vi "SetParam.vi"(8 "error in (no error)":errorcluster caption="entrée d'erreur (pas d'erreur)", 10 "KNNImputer":T1={"missing_values"="nan", "n_neighbors"=5, "weights"="uniform", "metric"="nan_euclidean", "copy"=TRUE, "add_indicator"=FALSE}, 11 "KNNImputer.lvclass":refnum<class "KNNImputer.lvclass">) -> (0 "error out":errorcluster caption="sortie d'erreur", 3 "KNNImputer.lvclass":refnum<class "KNNImputer.lvclass">)   [LabVIEW 2020, in "KNNImputer.lvclass"]
doc: "Set Parameters"
uses:
  KNNImputer.lvclass
  KNNImputer.lvclass/KNNImputer.ctl
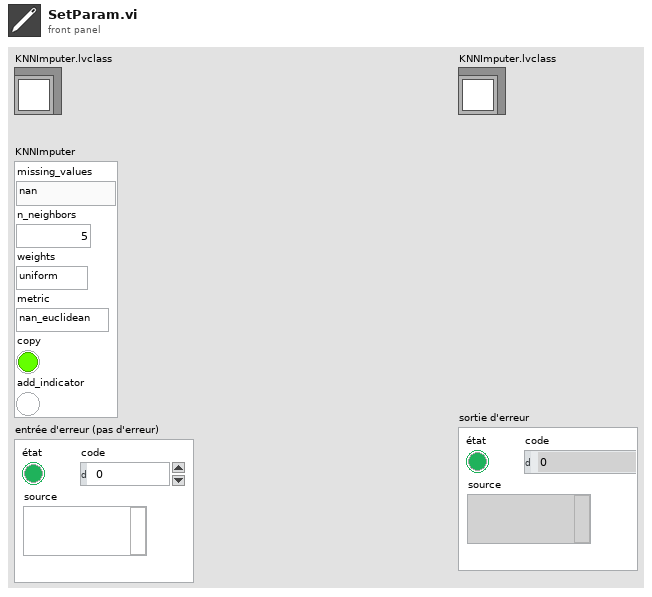
[diagram p1: front panel]
types:
  T1 = cluster{"missing_values":string, "n_neighbors":i32, "weights":string, "metric":string, "copy":bool, "add_indicator":bool}
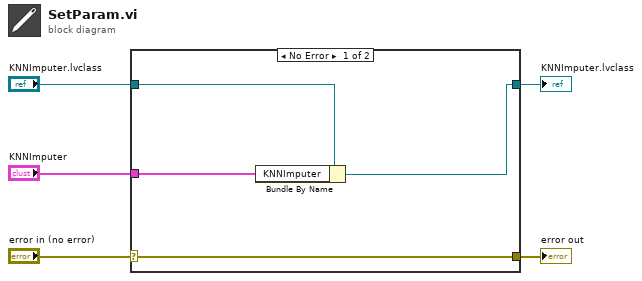
[diagram p0: block diagram]
diagram:
  n1 = case shown="No Error" "error in (no error)" {
    selector: "error in (no error)" -> [w9 w10]
    tunnel: [w9 w10] -> w4
    tunnel: [w7 w11] -> w2
    tunnel: "KNNImputer.lvclass" -> [w8 w11]
    tunnel: "KNNImputer" -> [w6 _]
    frame No Error {
      n2 = Bundle By Name(cluster=w8, "KNNImputer"=w6) -> (w7:refnum<class "KNNImputer.lvclass">)
    }
    frame Error {
    }
  }
  "error out" <- w4
  "KNNImputer.lvclass" <- w2
